vi "User Info.vi"(11 "URI in":refnum<class "URI.lvclass">) -> (1 "Password":string, 2 "Username":string, 3 "URI out":refnum<class "URI.lvclass">)   [LabVIEW 2020, in "URI.lvlib" / "URI.lvclass"]
uses:
  URI.lvclass
  URI.lvclass/URI.ctl
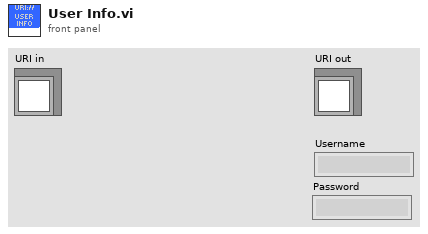
[diagram p1: front panel]
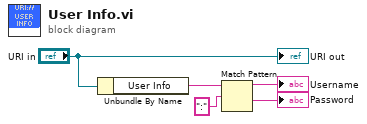
[diagram p0: block diagram]
diagram:
  n1 = Unbundle By Name("URI in") -> ("User Info"=w4:string)
  n2 = Match Pattern(string=w4, regular expression=":") -> (before substring=→"Username":string, after substring=→"Password":string)  [unwired: 1 in, 2 out]
  "URI out" <- "URI in"
